vi "PH_ImageOperator.Turn Image for Traces.vi"(0 "Operation Image":T1, 1 "Turn Image in":T1, 5 "error in (no error)":errorcluster) -> (8 "Major Offset":sgl, 10 "Major Trace":sgl[](array[numeric]) format="%.2f", 12 "Maj Dim":dbl, 15 "Minor Offset":sgl, 16 "Minor Trace":sgl[](array[numeric]) format="%.2f", 17 "Min Dim":dbl, 19 "error out":errorcluster)   [LabVIEW 2014, in "PH_ImageOperator.lvlib"]
doc: "This VI turns the \"Operation Image\" by the \"Turning Angle\" (by that, the image is copied to \"Turn Image\" not to change the \"Operation Image\"). The turned image is analyzed: the center of gravity traces (which are a column or row, resp. now) are given out."
uses:
  PH_ImageOperator.lvlib
  <vilib>/vision/Image Controls.llb/IMAQ Image.ctl
  <vilib>/vision/NI_Vision_Development_Module.lvlib
panel:
  in  "Turning Angle [rad]":dbl
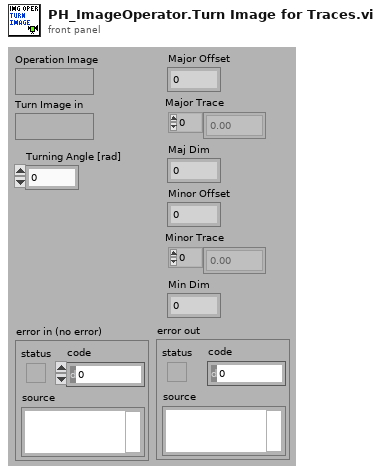
[diagram p1: front panel]
types:
  T1 = typedef "IMAQ Image.ctl" = refnum<image>
  T2 = typedef "PH_ImageOperator.lvlib/PH_ImageOperator.Beam Analysis Data.ctl" = cluster{"CoG-x":sgl, "CoG-y":sgl, "Maj Dim":dbl, "Min Dim":dbl, "Ellipticity":dbl, "Azimuth Angle [rad]":dbl, "Azi Angle rel to Maj?":bool}
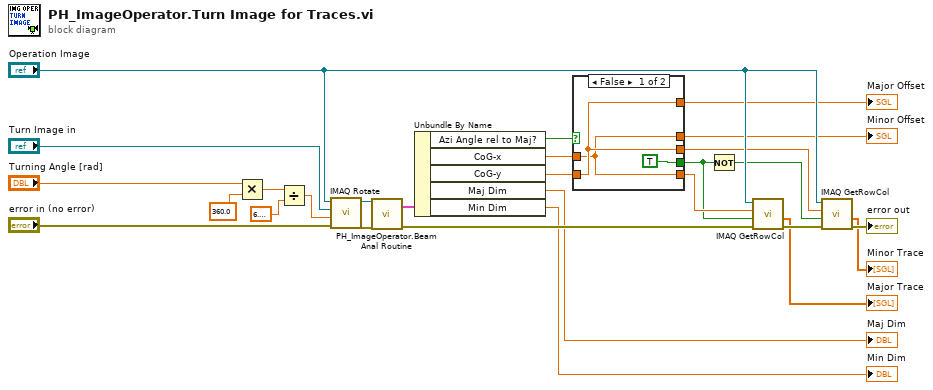
[diagram p0: block diagram]
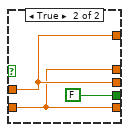
[diagram p2: hidden frame]
diagram:
  n1 = Multiply(x="Turning Angle [rad]", y=360.0) -> (x*y=w24:dbl)
  n2 = Divide(x=w24, y=6.283185307179586) -> (x/y=w22:dbl)
  n3 = call "IMAQ Rotate"("error in (no error)"="error in (no error)", "Angle (degrees)"=w22, "Image Dst"="Turn Image in", "Image Src"="Operation Image") -> ("error out"=w7:errorcluster, "Image Dst Out"=w5:T1)  [unwired: 6 in]
  n4 = call "PH_ImageOperator.Beam Anal Routine.vi"("Image"=w5, "error in (no error)"=w7) -> ("Analysis Data"=w4:T2, "error out"=w6:errorcluster)  [unwired: 13 in, 3 out]
  n5 = Unbundle By Name(w4) -> ("Azi Angle rel to Maj?"=w1:bool, "CoG-x"=w20:sgl, "CoG-y"=w21:sgl, "Maj Dim"=→"Maj Dim":dbl, "Min Dim"=→"Min Dim":dbl)
  n6 = case shown="False" w1 {
    tunnel: w21 -> [w29 w31]
    tunnel: w20 -> [w28 w32]
    tunnel: [w28 w31] -> w15
    tunnel: [TRUE FALSE] -> w14
    tunnel: [w29 w32] -> w12
    tunnel: [w29 w32] -> w10
    tunnel: [w28 w31] -> w9
    frame False {
    }
    frame True {
    }
  }
  "Major Offset" <- w10
  "Minor Offset" <- w9
  n7 = Not(x=w14) -> (.not. x?=w13:bool)
  n8 = call "IMAQ GetRowCol"("Image"="Operation Image", "Number"=w15, "Row / Column (Row)"=w14, "error in (no error)"=w6) -> ("Pixels (Float)"=→"Major Trace":sgl[], "error out"=w19:errorcluster)  [unwired: 2 in, 3 out]
  n9 = call "IMAQ GetRowCol"("Image"="Operation Image", "Number"=w12, "Row / Column (Row)"=w13, "error in (no error)"=w19) -> ("Pixels (Float)"=→"Minor Trace":sgl[], "error out"=→"error out":errorcluster)  [unwired: 2 in, 3 out]
